vi "Parse Config.vi"(7 "VolatusAPI":refnum<class "VolatusAPI.lvclass">, 8 "error in (no error)":errorcluster, 10 "Config Element":refnum<class "Config Element.lvclass">, 11 "GaugeIndicator in":refnum<class "GaugeIndicator.lvclass">) -> (0 "error out":errorcluster, 3 "GaugeIndicator out":refnum<class "GaugeIndicator.lvclass">)   [LabVIEW 2020, in "VolatusGUIElements.lvlib" / "GaugeIndicator.lvclass"]
uses:
  GaugeIndicator.lvclass
  lv-cdm/CDM-Config/Config Element/Config Element.lvclass
  Volatus/VolatusAPI/VolatusAPI.lvclass
  GaugeIndicator.lvclass/GaugeIndicator.ctl
  da521db5-3efc-46b7-b6a6-db04b27d7527.vi
  VolatusGUIElements.lvlib
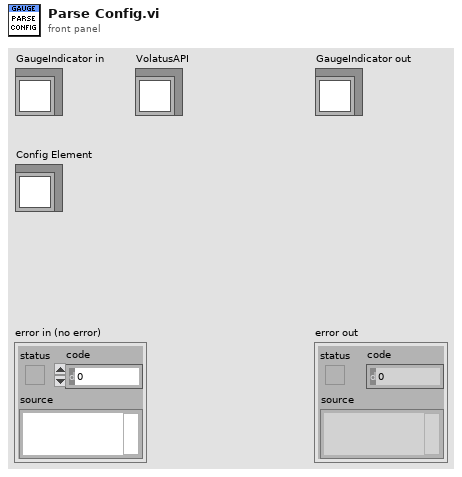
[diagram p1: front panel]
types:
  T1 = typedef "VolatusGUIElements.lvlib/GaugeIndicator.lvclass/Value Source.ctl" = enum16{"Constant", "Channel"}
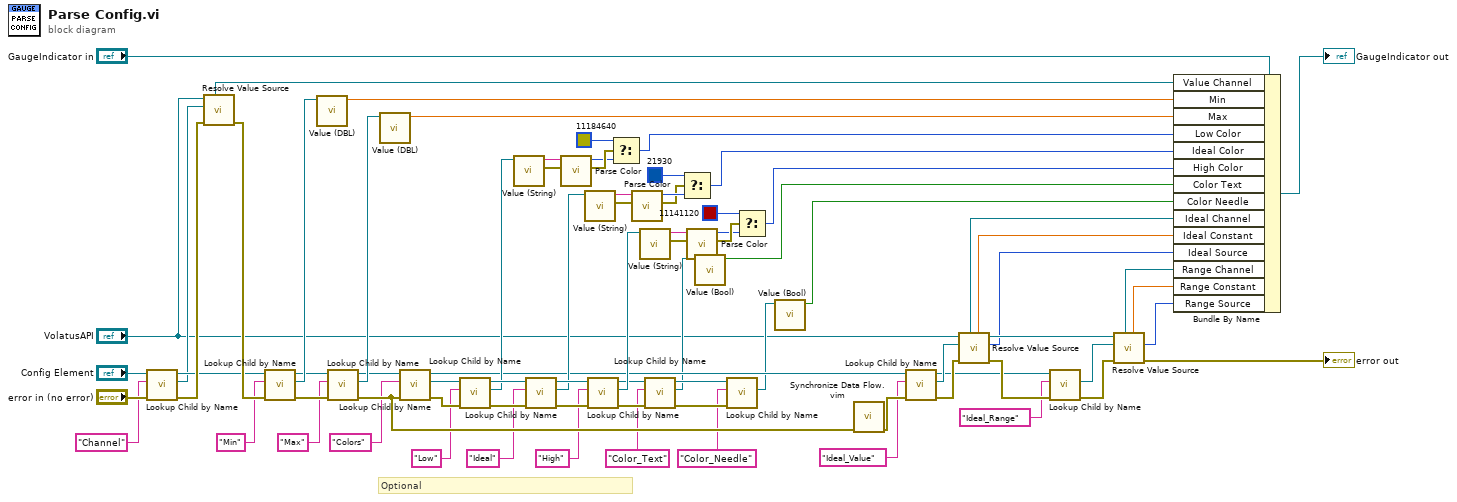
[diagram p0: block diagram]
diagram:
  # "Optional"
  n1 = call "Lookup Child by Name.vi"("error in (no error)"="error in (no error)", "Name"="Channel", "Config Element in"="Config Element") -> ("error out"=w79:errorcluster, "Child"=w3:refnum<class "Config Element.lvclass">, "Config Element out"=w63:refnum<class "Config Element.lvclass">)  [unwired: 5 in, 1 out]
  n2 = call "Resolve Value Source.vi"("error in (no error)"=w79, "Config Element"=w3, "VolatusAPI in"="VolatusAPI") -> ("error out"=w80:errorcluster, "Channel"=w1:refnum<class "Channel DBL.lvclass">)  [unwired: 4 in, 3 out]
  n3 = call "Lookup Child by Name.vi"("error in (no error)"=w80, "Name"="Min", "Config Element in"=w63) -> ("error out"=w70:errorcluster, "Child"=w62:refnum<class "Config Element.lvclass">, "Config Element out"=w58:refnum<class "Config Element.lvclass">)  [unwired: 5 in, 1 out]
  n4 = call "Value (DBL).vi"("Config Element in"=w62) -> ("DBL Value"=w61:dbl)  [unwired: 9 in, 1 out]
  n5 = call "Lookup Child by Name.vi"("error in (no error)"=w70, "Name"="Max", "Config Element in"=w58) -> ("error out"=w75:errorcluster, "Child"=w60:refnum<class "Config Element.lvclass">, "Config Element out"=w55:refnum<class "Config Element.lvclass">)  [unwired: 5 in, 1 out]
  n6 = call "Value (DBL).vi"("Config Element in"=w60) -> ("DBL Value"=w57:dbl)  [unwired: 9 in, 1 out]
  n7 = call "Lookup Child by Name.vi"("error in (no error)"=w75, "Name"="Colors", "Config Element in"=w55) -> ("error out"=w71:errorcluster, "Child"=w54:refnum<class "Config Element.lvclass">, "Config Element out"=w25:refnum<class "Config Element.lvclass">)  [unwired: 5 in, 1 out]
  n8 = call "Lookup Child by Name.vi"("error in (no error)"=w71, "Name"="Low", "Config Element in"=w54) -> ("error out"=w52:errorcluster, "Child"=w44:refnum<class "Config Element.lvclass">, "Config Element out"=w48:refnum<class "Config Element.lvclass">)  [unwired: 5 in, 1 out]
  n9 = call "Value (String).vi"("Config Element in"=w44) -> ("error out"=w45:errorcluster, "String Value"=w46:string)  [unwired: 9 in]
  n10 = call "Lookup Child by Name.vi"("error in (no error)"=w52, "Name"="Ideal", "Config Element in"=w48) -> ("error out"=w51:errorcluster, "Child"=w30:refnum<class "Config Element.lvclass">, "Config Element out"=w47:refnum<class "Config Element.lvclass">)  [unwired: 5 in, 1 out]
  n11 = call "Parse Color.vi"("error in (no error)"=w45, "Color String"=w46) -> ("error out"=w72:errorcluster, "Color"=w43:u32)  [unwired: 8 in]
  n12 = call "Value (String).vi"("Config Element in"=w30) -> ("error out"=w38:errorcluster, "String Value"=w37:string)  [unwired: 9 in]
  n13 = call "Lookup Child by Name.vi"("error in (no error)"=w51, "Name"="High", "Config Element in"=w47) -> ("error out"=w78:errorcluster, "Child"=w28:refnum<class "Config Element.lvclass">, "Config Element out"=w11:refnum<class "Config Element.lvclass">)  [unwired: 5 in, 1 out]
  n14 = Select(t=u32 11184640 ("color(black)"), s=w72, f=w43) -> (s? t:f=w41:u32)
  n15 = call "Parse Color.vi"("error in (no error)"=w38, "Color String"=w37) -> ("error out"=w36:errorcluster, "Color"=w39:u32)  [unwired: 8 in]
  n16 = call "Value (String).vi"("Config Element in"=w28) -> ("error out"=w33:errorcluster, "String Value"=w34:string)  [unwired: 9 in]
  n17 = call "Lookup Child by Name.vi"("error in (no error)"=w78, "Name"="Color_Text", "Config Element in"=w11) -> ("error out"=w77:errorcluster, "Child"=w7:refnum<class "Config Element.lvclass">, "Config Element out"=w8:refnum<class "Config Element.lvclass">)  [unwired: 5 in, 1 out]
  n18 = Select(t=u32 21930 ("color(black)"), s=w36, f=w39) -> (s? t:f=w29:u32)
  n19 = call "Parse Color.vi"("error in (no error)"=w33, "Color String"=w34) -> ("error out"=w35:errorcluster, "Color"=w32:u32)  [unwired: 8 in]
  n20 = call "Value (Bool).vi"("Config Element in"=w7) -> ("Bool Value"=w5:bool)  [unwired: 9 in, 1 out]
  n21 = call "Lookup Child by Name.vi"("error in (no error)"=w77, "Name"="Color_Needle", "Config Element in"=w8) -> ("Child"=w6:refnum<class "Config Element.lvclass">)  [unwired: 5 in, 3 out]
  n22 = Select(t=u32 11141120 ("color(black)"), s=w35, f=w32) -> (s? t:f=w27:u32)
  n23 = call "Value (Bool).vi"("Config Element in"=w6) -> ("Bool Value"=w4:bool)  [unwired: 9 in, 1 out]
  n24 = call "Synchronize Data Flow.vim"("input 4"=w75) -> ("output 4"=w76:errorcluster)  [unwired: 3 in, 3 out]
  n25 = call "Lookup Child by Name.vi"("error in (no error)"=w76, "Name"="Ideal_Value", "Config Element in"=w25) -> ("error out"=w73:errorcluster, "Child"=w23:refnum<class "Config Element.lvclass">, "Config Element out"=w20:refnum<class "Config Element.lvclass">)  [unwired: 5 in, 1 out]
  n26 = call "Resolve Value Source.vi"("error in (no error)"=w73, "Config Element"=w23, "VolatusAPI in"="VolatusAPI") -> ("error out"=w74:errorcluster, "Source"=w17:T1, "VolatusAPI"=w22:refnum<class "VolatusAPI.lvclass">, "Constant"=w18:dbl, "Channel"=w19:refnum<class "Channel DBL.lvclass">)  [unwired: 4 in]
  n27 = call "Lookup Child by Name.vi"("error in (no error)"=w74, "Name"="Ideal_Range", "Config Element in"=w20) -> ("error out"=w13:errorcluster, "Child"=w21:refnum<class "Config Element.lvclass">)  [unwired: 5 in, 2 out]
  n28 = call "Resolve Value Source.vi"("error in (no error)"=w13, "Config Element"=w21, "VolatusAPI in"=w22) -> ("error out"=→"error out":errorcluster, "Source"=w14:T1, "Constant"=w15:dbl, "Channel"=w16:refnum<class "Channel DBL.lvclass">)  [unwired: 4 in, 1 out]
  n29 = Bundle By Name(cluster="GaugeIndicator in", "Value Channel"=w1, "Min"=w61, "Max"=w57, "Low Color"=w41, "Ideal Color"=w29, "High Color"=w27, "Color Text"=w5, "Color Needle"=w4, "Ideal Channel"=w19, "Ideal Constant"=w18, "Ideal Source"=w17, "Range Channel"=w16, "Range Constant"=w15, "Range Source"=w14) -> (→"GaugeIndicator out":refnum<class "GaugeIndicator.lvclass">)
